vi "ReadWrite.EngineData.vi"(8 "error in":errorcluster, 11 "ReadWrite in":refnum<class "ReadWrite.lvclass">) -> (0 "error out":errorcluster, 3 "ReadWrite out":refnum<class "ReadWrite.lvclass">)   [LabVIEW 2015, in "Data Access API.lvlib" / "ReadWrite.lvclass"]
uses:
  ReadWrite.lvclass
  ReadWrite.lvclass/ReadWrite.ctl
  <vilib>/NI Veristand/Custom Device API/Global Data Refs.vi
  <vilib>/NI Veristand/Custom Device API/Custom Device API.lvlib
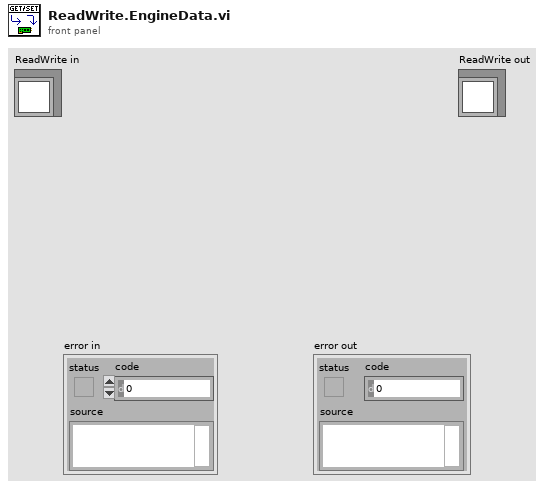
[diagram p1: front panel]
types:
  T1 = typedef "Custom Device API.lvlib/Data Reference.ctl" = i32
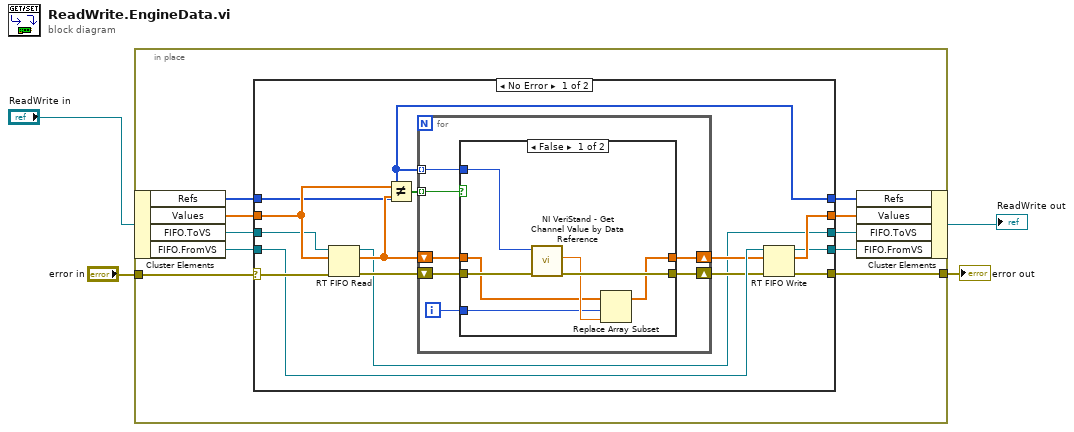
[diagram p0: block diagram]
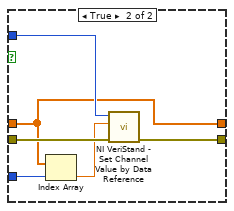
[diagram p2: hidden frame]
diagram:
  n1 = in-place {
    in-place-border: [w14] -> w4
    in-place-border: "error in" -> [w9]
    n2 = in-place-cluster #1("ReadWrite in") -> ("Refs"=w13:T1[], "Values"=w12:dbl[], "FIFO.ToVS"=w7:refnum<k33>, "FIFO.FromVS"=w8:refnum<k33>)
    n3 = case shown="No Error" w9 {
      selector: w9 -> [w25 w52]
      tunnel: [w27 w52] -> w14
      tunnel: [w18 w51] -> w11
      tunnel: w13 -> [w17 w50]
      tunnel: w12 -> [w24 w51]
      tunnel: [w17 w50] -> w10
      tunnel: w7 -> [w22 w49]
      tunnel: w8 -> [w21 w48]
      tunnel: [w15 w49] -> w6
      tunnel: [w16 w48] -> w5
      frame No Error {
        n4 = RT FIFO Read(0:w22, 1:w24, 3:w25) -> (8:w15:refnum<k33>, 9:w23:dbl[], 11:w26:errorcluster)  [unwired: 1 in, 2 out]
        n5 = Not Equal?(x=w24, y=w23) -> (x != y?=w20:bool[])
        n6 = for {
          shift-right: [w34] -> w19
          shift-left: w26 -> [w33]
          tunnel: w20 -> [w30] mode=indexing
          tunnel: w17 -> [w31] mode=indexing
          shift-right: [w28] -> w18
          shift-left: w23 -> [w32]
          i -> [w29]
          n7 = case shown="False" w30 {
            tunnel: w32 -> [w36 w42]
            tunnel: [w39 w46] -> w34
            tunnel: w33 -> [w40 w47]
            tunnel: w31 -> [w41 w45]
            tunnel: w29 -> [w37 w44]
            tunnel: [w35 w42] -> w28
            frame False {
              n8 = call <vilib>:"NI VeriStand - Get Channel Value by Data Reference.vi"("error in (no error)"=w40, "Data Reference in"=w41) -> ("error out"=w39:errorcluster, "Value"=w38:dbl)  [unwired: 8 in]
              n9 = Replace Array Subset(array=w36, new element=w38, index=w37) -> (w35:dbl[])
            }
            frame True {
              n10 = Index Array(array=w42, index=w44) -> (element=w43:dbl)
              n11 = call <vilib>:"NI VeriStand - Set Channel Value by Data Reference.vi"("error in (no error)"=w47, "Value"=w43, "Data Reference in"=w45) -> ("error out"=w46:errorcluster)  [unwired: 8 in]
            }
          }
        }
        n12 = RT FIFO Write(0:w21, 1:w18, 3:w19) -> (8:w16:refnum<k33>, 11:w27:errorcluster)  [unwired: 2 in, 2 out]
      }
      frame Error {
      }
    }
    n13 = in-place-cluster #1("Refs"=w10, "Values"=w11, "FIFO.ToVS"=w6, "FIFO.FromVS"=w5) -> (→"ReadWrite out":refnum<class "ReadWrite.lvclass">)
  }
  "error out" <- w4
